vi "SubSystems.vi"(8 "error in":errorcluster) -> ()   [LabVIEW 2018]
doc: "This VI calls the various robot subsystems that will then run in parallel. New subSystems will automatlically script code to make the call."
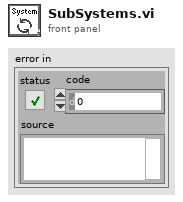
[diagram p1: front panel]
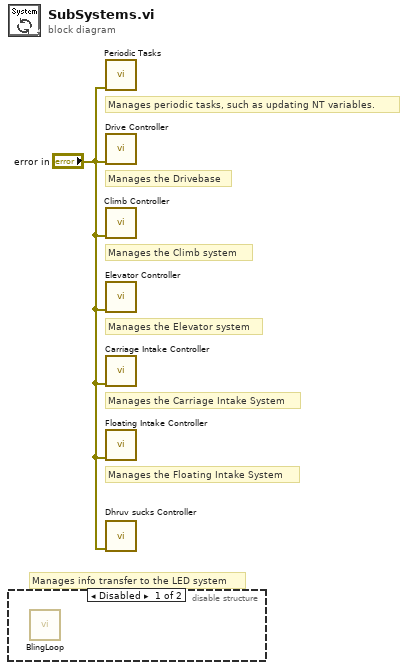
[diagram p0: block diagram]
diagram:
  # "Manages the Floating Intake System"
  # "Manages the Carriage Intake System"
  # "Manages the Elevator system"
  # "Manages the Climb system"
  # "Manages the Drivebase"
  # "Manages periodic tasks, such as updating NT variables."
  # "Manages info transfer to the LED system"
  n1 = disable-structure shown="Disabled" {
    frame Disabled {
      n2 = call "BlingLoop.vi"() -> ()  [unwired: 11 in, 1 out]
    }
    frame Enabled {
    }
  }
  n3 = call "Periodic Tasks.vi"("error in"="error in") -> ()  [unwired: 1 in, 10 out]
  n4 = call "Drive Controller.vi"("error in"="error in") -> ()  [unwired: 11 in]
  n5 = call "Climb Controller.vi"("error in"="error in") -> ()  [unwired: 11 in]
  n6 = call "Elevator Controller.vi"("error in"="error in") -> ()  [unwired: 11 in]
  n7 = call "Carriage Intake Controller.vi"("error in"="error in") -> ()  [unwired: 11 in]
  n8 = call "Floating Intake Controller.vi"("error in"="error in") -> ()  [unwired: 11 in]
  n9 = call "Dhruv sucks Controller.vi"("error in"="error in") -> ()  [unwired: 11 in]
